vi "Check Commands.vi"(8 "error in (no error)":refnum<class "MultiErrors.lvclass">, 11 "Sequence Validation in":refnum<class "Sequence Validation.lvclass">) -> (0 "error out":refnum<class "MultiErrors.lvclass">, 3 "Sequence Validation out":refnum<class "Sequence Validation.lvclass">)   [LabVIEW 2020, in "VolatusSeq.lvlib" / "Sequence Validation.lvclass"]
uses:
  Sequence Validation.lvclass
  VolatusErrorUtilities/MultiErrors/MultiErrors.lvclass
  Sequence Validation.lvclass/Sequence Validation.ctl
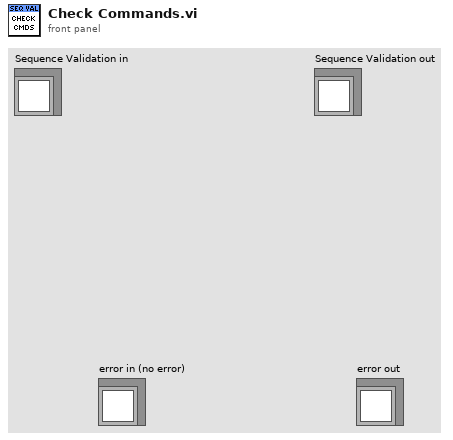
[diagram p1: front panel]
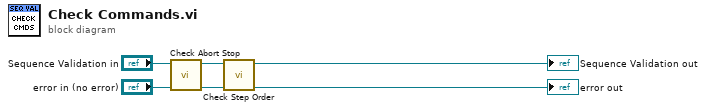
[diagram p0: block diagram]
diagram:
  n1 = call "Check Abort Stop.vi"("error in (no error)"="error in (no error)", "Sequence Validation in"="Sequence Validation in") -> ("error out"=w4:refnum<class "MultiErrors.lvclass">, "Sequence Validation out"=w3:refnum<class "Sequence Validation.lvclass">)  [unwired: 8 in]
  n2 = call "Check Step Order.vi"("error in (no error)"=w4, "Sequence Validation in"=w3) -> ("error out"=→"error out":refnum<class "MultiErrors.lvclass">, "Sequence Validation out"=→"Sequence Validation out":refnum<class "Sequence Validation.lvclass">)  [unwired: 8 in]
